vi "Anpassungspruefung.vi"(8 "Error in":errorcluster, 10 "Globale Variablen":T1, 11 "GUI Einstellungen":T2) -> (0 "Error out":errorcluster, 2 "Globale Variablen out":T1, 3 "GUI Einstellungen out":T2)   [LabVIEW 2016]
doc: "Weist nach der Flussdichte-Anpassung der Spannungsabweichung den minimal möglichen Spannungswert des Frequenzgenerators zu und stellt Spannung des Frequenzgenerators auf diesen Wert ein, wenn die Spannungsabweichung kleiner der minimal möglichen Spannung des Frequenzgenerators ist."
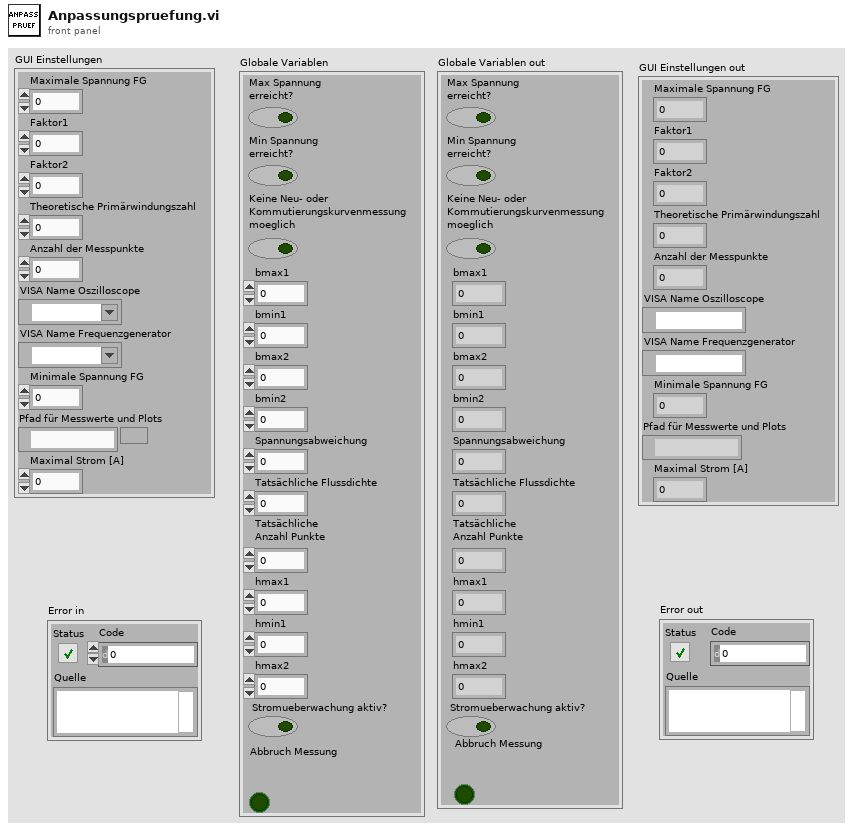
[diagram p1: front panel]
types:
  T1 = cluster{"Max Spannung\nerreicht?":bool, "Min Spannung\nerreicht?":bool, "Keine Neu- oder\nKommutierungskurvenmessung\nmoeglich":bool, "bmax1":dbl, "bmin1":dbl, "bmax2":dbl, "bmin2":dbl, "Spannungsabweichung":dbl, "Tatsächliche Flussdichte":dbl, "Tatsächliche \nAnzahl Punkte":dbl, "hmax1":dbl, "hmin1":dbl, "hmax2":dbl, " Stromueberwachung aktiv?":bool, "Abbruch Messung":bool}
  T2 = cluster{"Maximale Spannung FG":dbl, "Faktor1":dbl, "Faktor2":dbl, "Theoretische Primärwindungszahl":dbl, "Anzahl der Messpunkte":i32, "VISA Name Oszilloscope":refnum<visa-resource-name>, "VISA Name Frequenzgenerator":refnum<visa-resource-name>, "Minimale Spannung FG":dbl, "Pfad für Messwerte und Plots":path, "Maximal Strom [A] ":dbl}
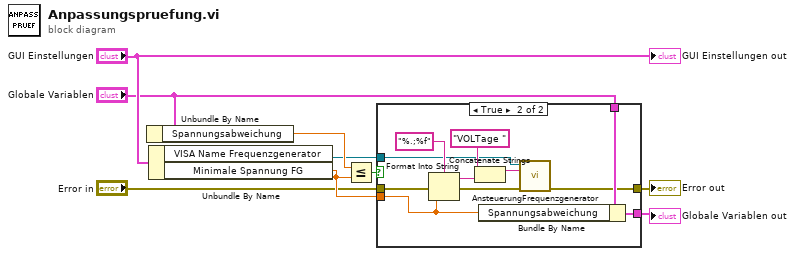
[diagram p0: block diagram]
diagram:
  n1 = Unbundle By Name("Globale Variablen") -> ("Spannungsabweichung"=w8:dbl)
  n2 = Unbundle By Name("GUI Einstellungen") -> ("VISA Name Frequenzgenerator"=w6:refnum<visa-resource-name>, "Minimale Spannung FG"=w7:dbl)
  n3 = Less Or Equal?(x=w8, y=w7) -> (x <= y?=w9:bool)
  n4 = case shown="True" w9 {
    tunnel: "Globale Variablen" -> [w10 w22]
    tunnel: [w10 w21] -> w1
    tunnel: w7 -> [_ w15]
    tunnel: w6 -> [_ w14]
    tunnel: "Error in" -> [w11 w13]
    tunnel: [w11 w12] -> w4
    frame False {
    }
    frame True {
      n5 = Format Into String(format string="%.;%f", error in=w13, w15) -> (resulting string=w18:string, error out=w19:errorcluster)  [unwired: 1 in]
      n6 = Concatenate Strings("VOLTage " ("String"), w18) -> (w17:string)
      n7 = Bundle By Name(cluster=w22, "Spannungsabweichung"=w15) -> (w21:T1)
      n8 = call "AnsteuerungFrequenzgenerator.vi"("Error_in"=w19, "Eingangs-String"=w17, "VISA Name FZ in(FZ)"=w14) -> ("Error_out"=w12:errorcluster)  [unwired: 5 in, 2 out]
    }
  }
  "Error out" <- w4
  "Globale Variablen out" <- w1
  "GUI Einstellungen out" <- "GUI Einstellungen"
